vi "外观模式DEMO.vi"() -> ()   [LabVIEW 2013]
uses:
  <vilib>/addons/_AddQ/G#Object/G#Object.lvclass
panel:
  out "Output":string
  out "# of objects killed":i32
  in  "停止":bool
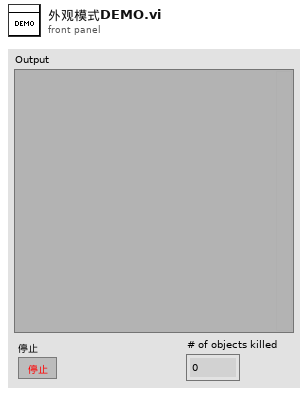
[diagram p1: front panel]
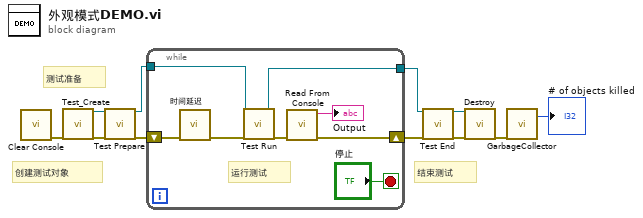
[diagram p0: block diagram]
diagram:
  # "结束测试"
  # "测试准备"
  # "创建测试对象"
  n1 = call "Clear Console.vi"() -> ("error out"=w1:errorcluster)  [unwired: 11 in]
  n2 = call "Test_Create.vi"("error in (no error)"=w1) -> ("reference out"=w11:refnum<class "Test.lvclass">, "error out"=w10:errorcluster)  [unwired: 17 in]
  n3 = call-dynamic "Test Prepare.vi"("reference in"=w11, "error in (no error)"=w10) -> ("reference out"=w8:refnum<class "Test.lvclass">, "error out"=w9:errorcluster)  [unwired: 16 in]
  n4 = while {
    shift-right: [w13] -> w6
    shift-left: w9 -> [w18]
    tunnel: w8 -> [w16]
    tunnel: [w15] -> w7
    stop <- "停止" stop-if-true
    # "运行测试"
    n5 = call "时间延迟"("error in (no error)"=w18) -> ("error out"=w17:errorcluster)  [unwired: 10 in]
    n6 = call-dynamic "Test Run.vi"("reference in"=w16, "error in (no error)"=w17) -> ("reference out"=w15:refnum<class "Test.lvclass">, "error out"=w14:errorcluster)  [unwired: 16 in]
    n7 = call "Read From Console.vi"("error in (no error)"=w14) -> ("error out"=w13:errorcluster, "Output"=→"Output":string)  [unwired: 9 in]
  }
  n8 = call-dynamic "Test End.vi"("reference in"=w7, "error in (no error)"=w6) -> ("reference out"=w4:refnum<class "Test.lvclass">, "error out"=w5:errorcluster)  [unwired: 16 in]
  n9 = call-dynamic "Destroy.vi"("reference in"=w4, "error in (no error)"=w5) -> ("error out"=w3:errorcluster)  [unwired: 16 in, 1 out]
  n10 = call <vilib>:"GarbageCollector.vi"("error in (no error)"=w3) -> ("# of objects killed"=→"# of objects killed":i32)  [unwired: 16 in, 2 out]
